vi "updateTextIcon.vi"(8 "error in (no error)":errorcluster, 9 "Text":T1, 10 "vi refnum":refnum<vi>, 11 "VirtualInstrument in":refnum<class "VirtualInstrument.lvclass">) -> (0 "error out":errorcluster, 2 "vi refnum 2":refnum<vi>, 3 "VirtualInstrument out":refnum<class "VirtualInstrument.lvclass">)   [LabVIEW 2013, in "VirtualInstrument.lvclass"]
uses:
  VirtualInstrument.lvclass
  <vilib>/LabVIEW Icon API/API_Text.ctl
  <vilib>/LabVIEW Icon API/API_Test Settings.ctl
  <vilib>/LabVIEW Icon API/lv_icon/Controls/Alignment.ctl
  <vilib>/LabVIEW Icon API/API_Text Colors.ctl
  <vilib>/LabVIEW Icon API/LabVIEW Icon API.lvlib
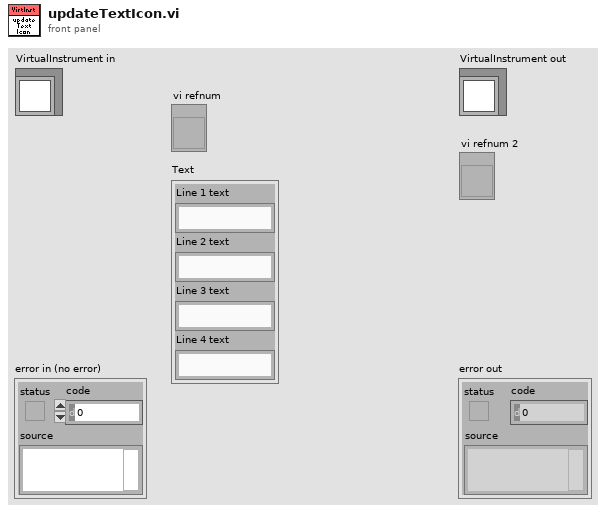
[diagram p1: front panel]
types:
  T1 = typedef "LabVIEW Icon API.lvlib/API_Text.ctl" = cluster{"Line 1 text":string, "Line 2 text":string, "Line 3 text":string, "Line 4 text":string}
  T2 = typedef "LabVIEW Icon API.lvlib/API_Test Settings.ctl" = cluster{"Font":string, "Alignment":T3, "Size":u8, "Center text":bool, "Capitalize text":bool, "Text color":T4}
  T3 = typedef "Alignment.ctl" = u16
  T4 = typedef "LabVIEW Icon API.lvlib/API_Text Colors.ctl" = cluster{"Line 1 color":u32, "Line 2 color":u32, "Line 3 color":u32, "Line 4 color":u32}
  T5 = typedef "LabVIEW Icon API.lvlib/API_User Layer Data.ctl" = cluster{"Layer name":string, "Origin":T6, "Icon image data":T7}
  T6 = typedef "LVPoint32TypeDef.ctl" = cluster{"Horizontal":i32, "Vertical":i32}
  T7 = typedef "imagedata.ctl" = cluster{"image type":i32, "image depth":i32, "image":u8[], "mask":u8[], "colors":u32[], "Rectangle":cluster{"left":i16, "top":i16, "right":i16, "bottom":i16}}
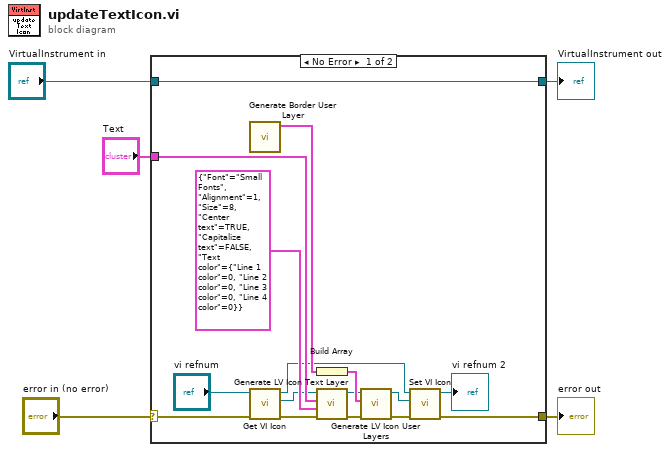
[diagram p0: block diagram]
diagram:
  n1 = case shown="No Error" "error in (no error)" {
    selector: "error in (no error)" -> [w7 w23]
    tunnel: [w6 w23] -> w4
    tunnel: [w21 w22] -> w2
    tunnel: "VirtualInstrument in" -> [w21 w22]
    tunnel: "Text" -> [w15 _]
    frame No Error {
      n2 = call <vilib>:"Generate Border User Layer.vi"() -> ("User Layer data"=w16:T5)  [unwired: 11 in]
      n3 = call <vilib>:"Get VI Icon.vi"("error in (no error)"=w7, "VI Refnum in"="vi refnum") -> ("error out"=w8:errorcluster, "Icon"=w13:refnum<class "Icon.lvclass">, "VI Refnum out"=w10:refnum<vi>)  [unwired: 7 in]
      n4 = Build Array(w16) -> (w12:T5[])
      n5 = call <vilib>:"Generate LV Icon Text Layer.vi"("error in (no error)"=w8, "Text settings"=T2 {"Font"="Small Fonts", "Alignment"=1, "Size"=8, "Center text"=TRUE, "Capitalize text"=FALSE, "Text color"={"Line 1 color"=0, "Line 2 color"=0, "Line 3 color"=0, "Line 4 color"=0}}, "Text"=w15, "Icon in"=w13) -> ("error out"=w19:errorcluster, "Icon out"=w11:refnum<class "Icon.lvclass">)  [unwired: 6 in]
      n6 = call <vilib>:"Generate LV Icon User Layers.vi"("error in (no error)"=w19, "User layers"=w12, "Icon in"=w11) -> ("error out"=w17:errorcluster, "Icon out"=w18:refnum<class "Icon.lvclass">)  [unwired: 7 in]
      n7 = call <vilib>:"Set VI Icon.vi"("error in (no error)"=w17, "Icon"=w18, "VI Refnum in"=w10) -> ("error out"=w6:errorcluster, "VI Refnum out"=→"vi refnum 2":refnum<vi>)  [unwired: 7 in]
    }
    frame Error {
    }
  }
  "error out" <- w4
  "VirtualInstrument out" <- w2
